vi "Open VISA Session Monitor.vi"() -> ()   [LabVIEW 2019]
panel:
  out "Actual Update":dbl format="%.3g"
  in  "Update Time (S)":dbl=0.25 format="%.3g"
  out "Number of\nOpen Sessions":dbl
  in  "Stop Button":bool
  in  "Remove Button":bool
  in  "Cancel Button":bool
  in  "Select All":bool
  in  "Current Open Sessions":i32[](listbox)
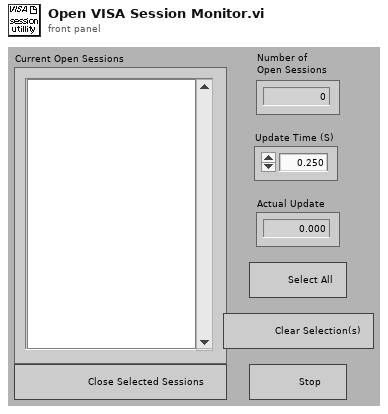
[diagram p1: front panel]
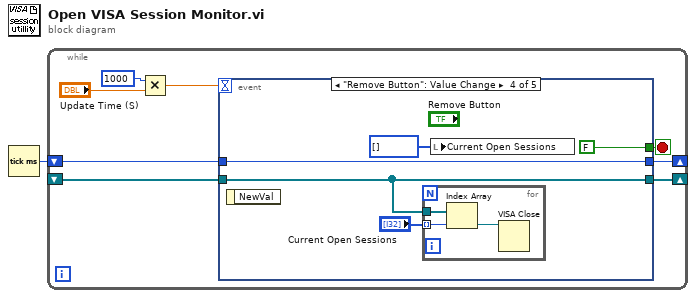
[diagram p0: block diagram]
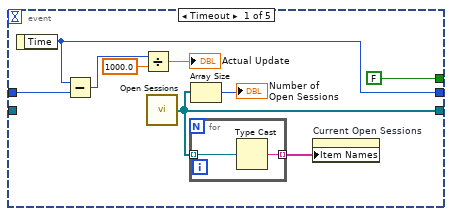
[diagram p2: hidden frame]
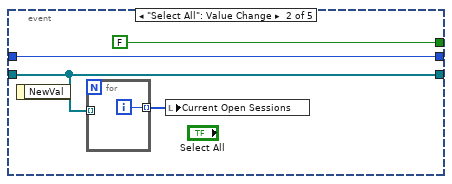
[diagram p3: hidden frame]
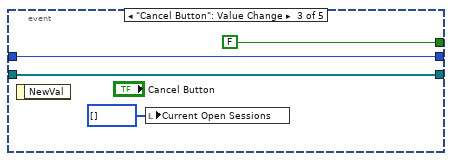
[diagram p4: hidden frame]
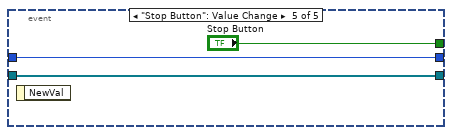
[diagram p5: hidden frame]
diagram:
  n1 = Tick Count (ms)() -> (millisecond timer value=w1:u32)
  n2 = while {
    shift-right: [w5] -> _
    shift-left: w1 -> [w6]
    shift-right: [w3] -> _
    shift-left: _ -> [w2]
    stop <- w4 stop-if-true
    n3 = Multiply(x=u32 1000 ("milliseconds to wait"), y="Update Time (S)") -> (x*y=w7:dbl)
    n4 = event shown="[3] \"Remove Button\": Value Change" {
      selector: _ -> [_ _ _ _ _]
      dyn-events: _ -> [_ _ _ _ _]
      timeout: w7 -> [_ _ _ _ _]
      tunnel: w6 -> [w15 w22 w27 w31 w38]
      tunnel: [w14 w22 w27 w31 w38] -> w5
      tunnel: [FALSE ("Quit") FALSE ("Quit") FALSE ("Quit") FALSE ("Quit") "Stop Button"] -> w4
      tunnel: [w11 w23 w26 w32 w39] -> w3
      tunnel: w2 -> [_ w23 w26 w32 w39]
      event Timeout {
        n5 = event-data() -> ("Time"=w14:u32)  [unwired: 1 in]
        n6 = Subtract(x=w14, y=w15) -> (x-y=w16:u32)
        n7 = Divide(x=w16, y=1000.0 ("Actual Update (s)")) -> (x/y=→"Actual Update":dbl)
        n8 = call <vilib>:"Open Sessions.vi"() -> ("Array of Refnums"=w11:refnum<visa-resource-name>[])  [unwired: 2 in]
        n9 = for {
          tunnel: w11 -> [w20] mode=indexing
          tunnel: [w19] -> w13 mode=indexing
          n10 = Type Cast(x=w20) -> (*(type *) &x=w19:string)  [unwired: 1 in]
        }
        n11 = Array Size(array=w11) -> (size(s)=→"Number of\nOpen Sessions":i32)
        n12 = property on="Current Open Sessions" class="LstBox (strict)"("Item Names"=w13) -> ()  [unwired: 2 in, 2 out]
      }
      event "Select All": Value Change {
        n13 = event-data() -> ()  [unwired: 1 in, 1 out]
        n14 = for {
          tunnel: [w25] -> w24 mode=indexing
          tunnel: w23 -> [_] mode=indexing
          i -> [w25]
        }
        n15 = local write "Current Open Sessions"(w24) -> ()
      }
      event "Cancel Button": Value Change {
        n16 = event-data() -> ()  [unwired: 1 in, 1 out]
        n17 = local write "Current Open Sessions"(i32[] [] ("Open sessions")) -> ()
      }
      event "Remove Button": Value Change {
        n18 = event-data() -> ()  [unwired: 1 in, 1 out]
        n19 = for {
          tunnel: w32 -> [w35]
          tunnel: "Current Open Sessions" -> [w37] mode=indexing
          n20 = Index Array(array=w35, index=w37) -> (element=w36:refnum<visa-resource-name>)
          n21 = VISA Close(VISA resource name=w36) -> ()  [unwired: 1 in, 1 out]
        }
        n22 = local write "Current Open Sessions"(i32[] [] ("Open sessions")) -> ()
      }
      event "Stop Button": Value Change {
        n23 = event-data() -> ()  [unwired: 1 in, 1 out]
      }
    }
  }
